vi "X-_Configure.vi"(0 "Address":u8, 1 "Port Name":string, 2 "Static Drive Configuration":T1={"Correction Gain % (CG)"=1, "Dead Band (DB)"=10, "Dead Band Window (DW)"=10, "Encoder Resolution (ER)"=4000, "Step Mode  (FSB)"=0, "Position Maintenance (FSC)"=0, "Stop on Stall (FSD)"=0, "Activate OP1 on stall (FSE)"=0, "Stop on Trigger 3 (FSF)"=0, "OP2 in Deadband (FSG)"=0, "Stall Detect (FSH)"=0, "Limit Disable (LD)"=0, "Motor Resolution (MR)"=enum."20000", "Limit Switch Sense (OSA)"=0, "Home Position (OSB)"=1, "Home Switch Sense (OSC)"=0, "Encoder Z for Home (OSD)"=0, "Reference edge of Home (OSH)"=0, "RS232 Echo Control (SSA)"=0, "Buffer at Limit (SSG)"=1, "Buffer at Stop (SSH)"=1, "Indexer Mode  (FSA)"=1, "Type"="", "ConfigString"="", "De Power Motor"=enum."FALSE"} {"Indexer Mode  (FSA)" items=["Incremental", "Absolute"]; "Buffer at Stop (SSH)" items=["Clear buffer", "Save and Continue"]; "Buffer at Limit (SSG)" items=["Clear buffer", "Save and Continue"]; "RS232 Echo Control (SSA)" items=["Echo ON", "Echo OFF"]; "Reference edge of Home (OSH)" items=["CW", "CCW"]; "Encoder Z for Home (OSD)" items=["Don't use", "Enable"]; "Home Switch Sense (OSC)" items=["Normally Open", "Normally Closed"]; "Home Position (OSB)" items=["Anywhere in Switch", "Edge of Switch"]; "Limit Switch Sense (OSA)" items=["Normally Closed", "Normally Open"]; "Limit Disable (LD)" items=["Both Enabled", "CW Disabled", "CCW Disabled", "Both Disabled"]; "Stall Detect (FSH)" items=["Disable", "Enable"]; "OP2 in Deadband (FSG)" items=["Don't Use", "ACTIVATE"]; "Stop on Trigger 3 (FSF)" items=["Ignore", "STOP!"]; "Activate OP1 on stall (FSE)" items=["Do not Activate", "ACTIVATE!"]; "Stop on Stall (FSD)" items=["Continue", "STOP"]; "Position Maintenance (FSC)" items=["Disabled", "Enabled"]; "Step Mode  (FSB)" items=["Motor", "Encoder"]; "Encoder Resolution (ER)" min=1 max=50000; "Dead Band Window (DW)" min=0 max=999999999; "Dead Band (DB)" min=0 max=999999999; "Correction Gain % (CG)" items=["n/a", "12.5", "25", "37.5", "50", "62.5", "75", "87.5", "100"]}, 3 "Channel Name":string) -> (8 "Good Echo":bool)   [LabVIEW 2010]
uses:
  ~subVIs/DriveStaticConfig.ctl
panel:
  out "Sent":string[](array[string])
  out "x = y?":bool[](array[boolean])
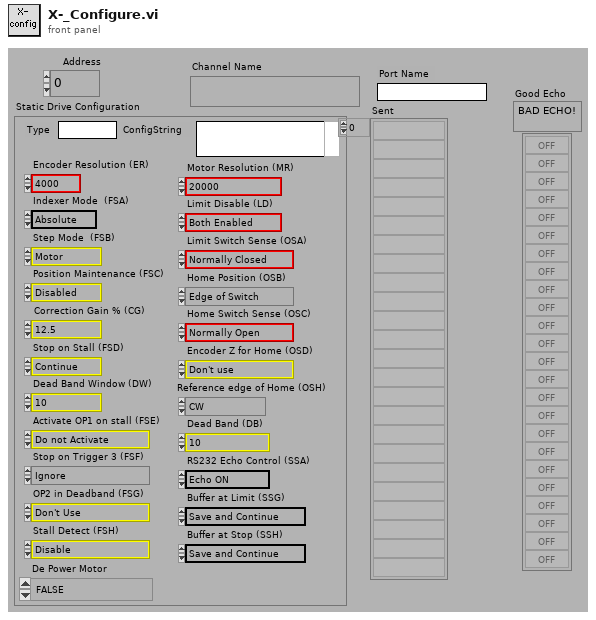
[diagram p1: front panel]
types:
  T1 = typedef "DriveStaticConfig.ctl" = cluster{"Correction Gain % (CG)":u16, "Dead Band (DB)":i32, "Dead Band Window (DW)":i32, "Encoder Resolution (ER)":i32, "Step Mode  (FSB)":u16, "Position Maintenance (FSC)":u16, "Stop on Stall (FSD)":u16, "Activate OP1 on stall (FSE)":u16, "Stop on Trigger 3 (FSF)":u16, "OP2 in Deadband (FSG)":u16, "Stall Detect (FSH)":u16, "Limit Disable (LD)":u16, "Motor Resolution (MR)":enum16{"200", "400", "1000", "2000", "4000", "5000", "10000", "12800", "18000", "20000", "21600", "25000", "25400", "25600", "36000", "50000", "278528", "425984", "507904", "614400", "655360", "819200", "1024000"}, "Limit Switch Sense (OSA)":u16, "Home Position (OSB)":u16, "Home Switch Sense (OSC)":u16, "Encoder Z for Home (OSD)":u16, "Reference edge of Home (OSH)":u16, "RS232 Echo Control (SSA)":u16, "Buffer at Limit (SSG)":u16, "Buffer at Stop (SSH)":u16, "Indexer Mode  (FSA)":u16, "Type":string, "ConfigString":string, "De Power Motor":enum16{"TRUE", "FALSE"}}
  T2 = enum16{"200", "400", "1000", "2000", "4000", "5000", "10000", "12800", "18000", "20000", "21600", "25000", "25400", "25600", "36000", "50000", "278528", "425984", "507904", "614400", "655360", "819200", "1024000"}
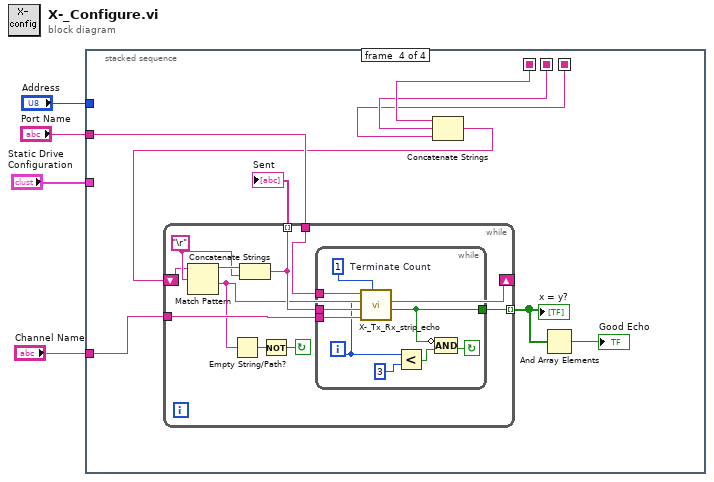
[diagram p0: block diagram]
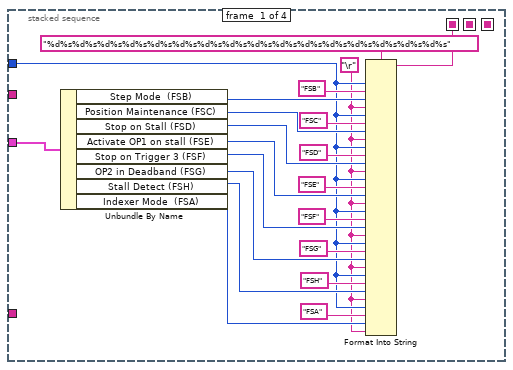
[diagram p2: hidden frame]
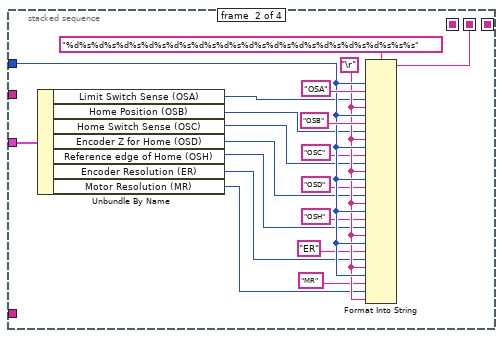
[diagram p3: hidden frame]
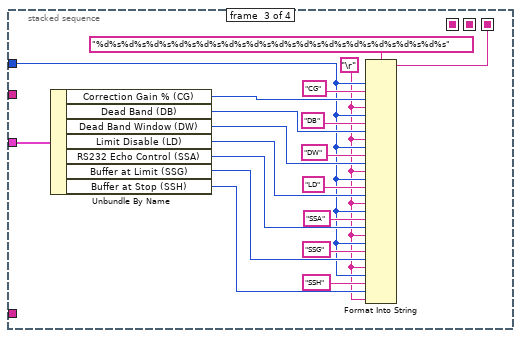
[diagram p4: hidden frame]
diagram:
  n1 = stacked-sequence {
    seq-local: [w24 _ _ _] -> [_ _ _ w72]
    seq-local: [_ w26 _ _] -> [_ _ _ w71]
    seq-local: [_ _ w51 _] -> [_ _ _ w70]
    tunnel: "Static Drive Configuration" -> [w25 w34 w58 _]
    tunnel: "Address" -> [w8 w42 w46 _]
    tunnel: "Port Name" -> [_ _ _ w69]
    tunnel: "Channel Name" -> [_ _ _ w67]
    frame #0 {
      w5 = "\r"
      n2 = Unbundle By Name(w25) -> ("Step Mode  (FSB)"=w22:u16, "Position Maintenance (FSC)"=w20:u16, "Stop on Stall (FSD)"=w14:u16, "Activate OP1 on stall (FSE)"=w13:u16, "Stop on Trigger 3 (FSF)"=w12:u16, "OP2 in Deadband (FSG)"=w11:u16, "Stall Detect (FSH)"=w10:u16, "Indexer Mode  (FSA)"=w6:u16)
      n3 = Format Into String(format string="%d%s%d%s%d%s%d%s%d%s%d%s%d%s%d%s%d%s%d%s%d%s%d%s%d%s%d%s%d%s%d%s", w8, "FSB", w22, w5, w8, "FSC", w20, w5, w8, "FSD", w14, w5, w8, "FSE", w13, w5, w8, "FSF", w12, w5, w8, "FSG", w11, w5, w8, "FSH", w10, w5, w8, "FSA", w6, w5) -> (resulting string=w24:string)  [unwired: 2 in, 1 out]
    }
    frame #1 {
      w41 = "\r"
      n4 = Unbundle By Name(w34) -> ("Limit Switch Sense (OSA)"=w33:u16, "Home Position (OSB)"=w32:u16, "Home Switch Sense (OSC)"=w31:u16, "Encoder Z for Home (OSD)"=w30:u16, "Reference edge of Home (OSH)"=w29:u16, "Encoder Resolution (ER)"=w28:i32, "Motor Resolution (MR)"=w27:T2)
      n5 = Format Into String(format string="%d%s%d%s%d%s%d%s%d%s%d%s%d%s%d%s%d%s%d%s%d%s%d%s%d%s%s%s", w42, "OSA", w33, w41, w42, "OSB", w32, w41, w42, "OSC", w31, w41, w42, "OSD", w30, w41, w42, "OSH", w29, w41, w42, "ER", w28, w41, w42, "MR", w27, w41) -> (resulting string=w26:string)  [unwired: 2 in, 1 out]
    }
    frame #2 {
      w45 = "\r"
      n6 = Unbundle By Name(w58) -> ("Correction Gain % (CG)"=w57:u16, "Dead Band (DB)"=w56:i32, "Dead Band Window (DW)"=w55:i32, "Limit Disable (LD)"=w54:u16, "RS232 Echo Control (SSA)"=w47:u16, "Buffer at Limit (SSG)"=w53:u16, "Buffer at Stop (SSH)"=w52:u16)
      n7 = Format Into String(format string="%d%s%d%s%d%s%d%s%d%s%d%s%d%s%d%s%d%s%d%s%d%s%d%s%d%s%d%s", w46, "CG", w57, w45, w46, "DB", w56, w45, w46, "DW", w55, w45, w46, "LD", w54, w45, w46, "SSA", w47, w45, w46, "SSG", w53, w45, w46, "SSH", w52, w45) -> (resulting string=w51:string)  [unwired: 2 in, 1 out]
    }
    frame #3 {
      n8 = Concatenate Strings(w72, w71, w70) -> (w64:string)
      n9 = while {
        tunnel: [w77] -> w66 mode=indexing
        tunnel: w67 -> [w78]
        tunnel: [w81] -> w68 mode=indexing
        tunnel: w69 -> [w79]
        shift-left: w64 -> [w76]
        shift-right: [w75] -> _
        stop <- w73 continue-if-true
        w80 = "\r"
        n10 = Match Pattern(string=w76, regular expression=w80) -> (before substring=w82:string, after substring=w75:string)  [unwired: 1 in, 2 out]
        n11 = Empty String/Path?(string/path=w75) -> (empty?=w74:bool)
        n12 = Concatenate Strings(w82, w80) -> (w81:string)
        n13 = Not(x=w74) -> (.not. x?=w73:bool)
        n14 = while {
          tunnel: [w84] -> w77
          tunnel: w78 -> [w89]
          tunnel: w79 -> [w90]
          tunnel: w81 -> [w91]
          i -> [w85]
          stop <- w86 continue-if-true
          w83 = 1  # Terminate Count
          n15 = call "X-_Tx_Rx_strip_echo.vi"("Terminate Count"=w83, "Channel Name"=w89, "Write String"=w91, "Iteration No"=w85, "Port Name"=w90) -> ("Good Echo"=w84:bool)  [unwired: 1 in, 2 out]
          n16 = Less?(x=w85, y=3) -> (x < y?=w87:bool)
          n17 = Compound Arithmetic op=AND(invert w84, w87) -> (w86:bool)
        }
      }
      "Sent" <- w68
      "x = y?" <- w66
      n18 = And Array Elements(Boolean array=w66) -> (logical AND=→"Good Echo":bool)
    }
  }
